vi "VAJ sim.vi"() -> ()   [LabVIEW 2019]
uses:
  <vilib>/Platform/TimedLoop/XDataNode/timing_clust.ctl
  <vilib>/Platform/TimedLoop/XDataNode/nitl_modes.ctl
  <vilib>/Platform/TimedLoop/XDataNode/wakeup.ctl
  <vilib>/platform/TimedLoop/XDataNode/XDataNode.xnode
  <vilib>/Platform/TimedLoop/XDataNode/XDNodeRunTimeDep.lvlib
panel:
  out "Waveform Chart":T1(graph)
  in  "D":dbl
  in  "J":dbl
  in  "A":dbl
  in  "V":dbl
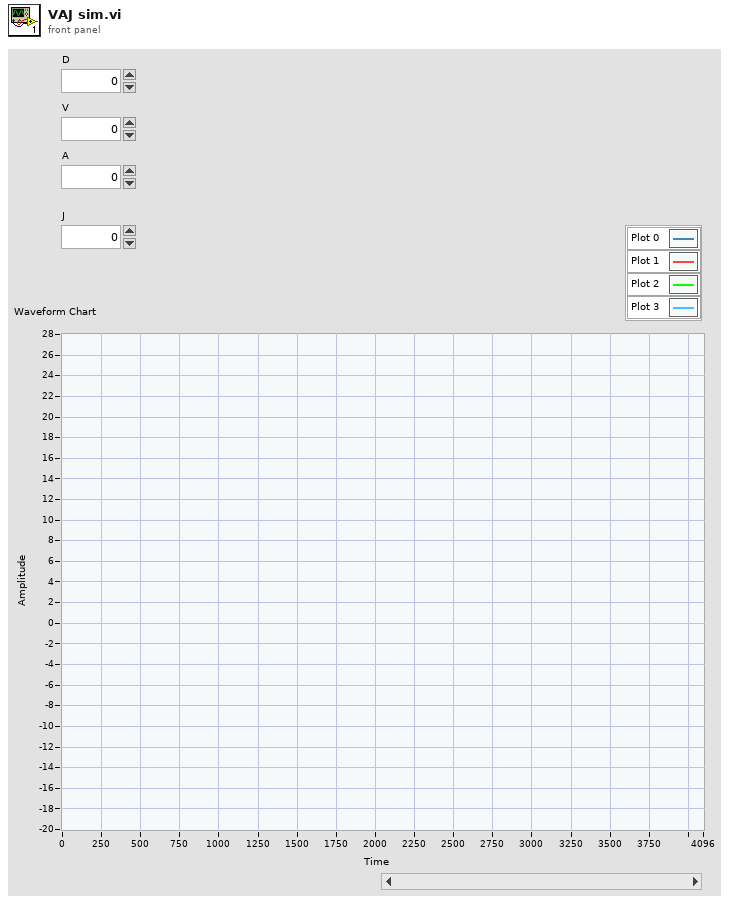
[diagram p1: front panel]
types:
  T1 = cluster{"setpoint":dbl, "integral x(t)":dbl, "integral x(t)":dbl, "integral x(t)":dbl}
  T2 = typedef "XDNodeRunTimeDep.lvlib/timing_clust.ctl" = cluster{"Expected End [f-1]":u64, "Actual End [f-1]":u64, "Finished Late? [f-1]":bool, "Expected End [i-1]":u64, "Actual End [i-1]":u64, "Finished Late? [i-1]":bool, "Expected Start [i]":u64, "Actual Start [i]":u64, "Expected Start [f]":u64, "Actual Start [f]":u64, "Source Name":string, "Structure Name":string, "Period":i64, "Deadline":i64, "Offset":i64, "Start":i64, "Priority":i32, "Timeout":i32, "Mode":T3, "Wakeup Reason":T4, "Error":errorcluster, "Source Type":string, "Secondary Source Type":string, "Global End Time":u64, "Global Start Time":u64, "Frame Duration":u64, "Iteration Duration":u64, "Assigned CPU":i32, "I/O Scan Engine Mode":u32}
  T3 = typedef "XDNodeRunTimeDep.lvlib/nitl_modes.ctl" = enum32{"No Change", "Process missed periods, maintain original phase", "Discard missed periods, maintain original phase", "Process missed periods, ignore original phase", "Discard missed periods, ignore original phase"}
  T4 = typedef "XDNodeRunTimeDep.lvlib/wakeup.ctl" = enum32{"Normal", "Aborted", "Asynchronous wakeup", "Timing source error", "Timed loop error", "Timeout"}
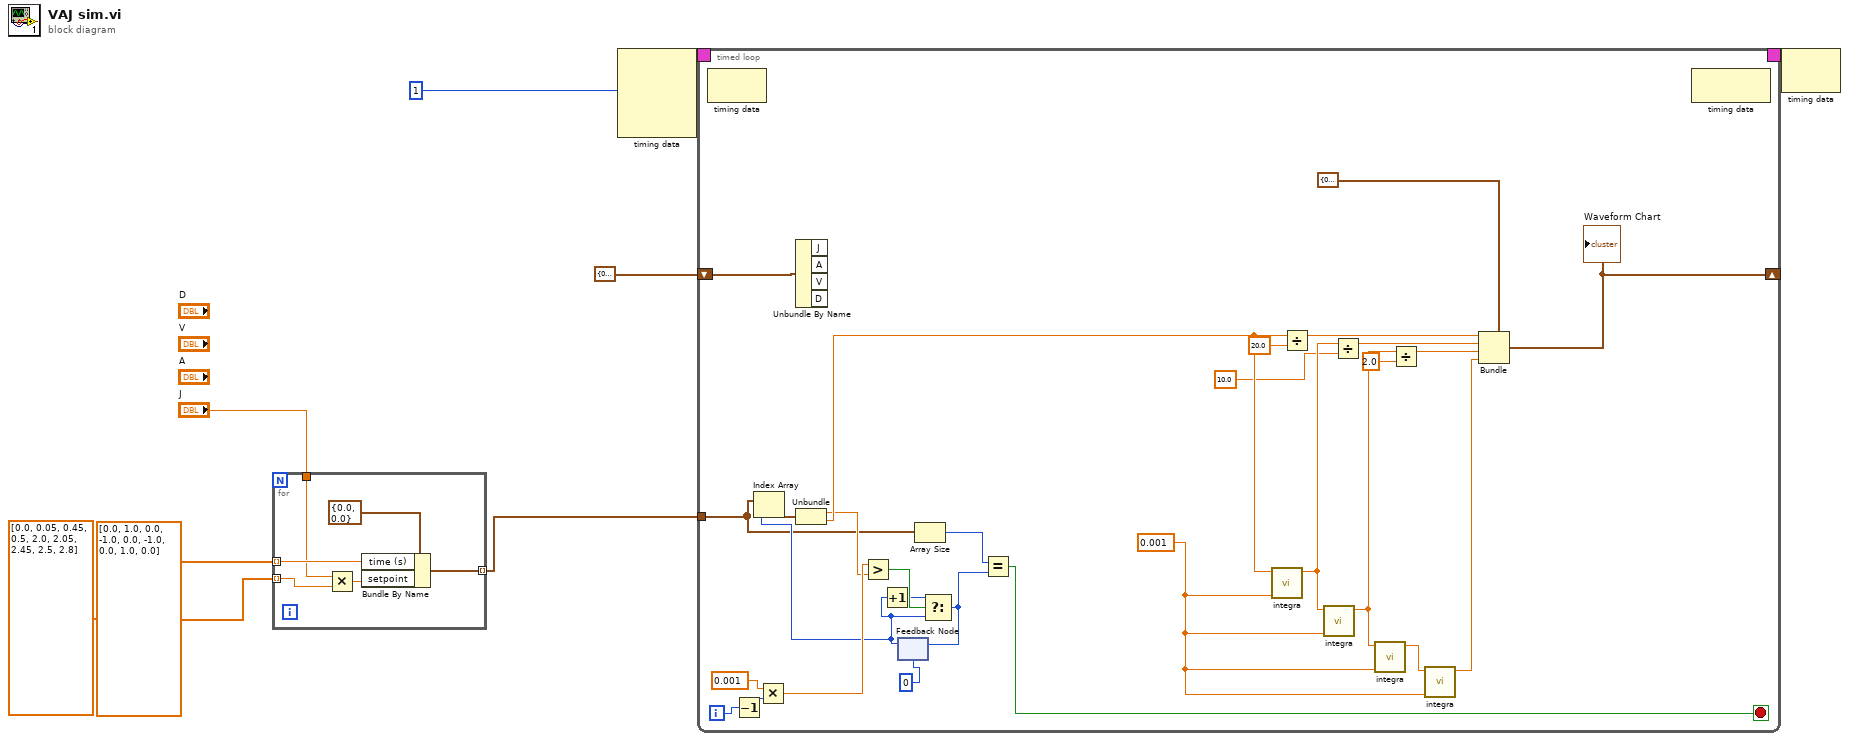
[diagram p0: block diagram]
diagram:
  n1 = for {
    tunnel: dbl[] [0.0, 0.05, 0.45, 0.5, 2.0, 2.05, 2.45, 2.5, 2.8] ("time (s)") -> [w13] mode=indexing
    tunnel: dbl[] [0.0, 1.0, 0.0, -1.0, 0.0, -1.0, 0.0, 1.0, 0.0] ("time (s)") -> [w9] mode=indexing
    tunnel: [w12] -> w3 mode=indexing
    tunnel: "J" -> [w10]
    n2 = Multiply(x=w10, y=w9) -> (x*y=w11:dbl)
    n3 = Bundle By Name(cluster=cluster{"time (s)":dbl, "setpoint":dbl} {"time (s)"=0.0, "setpoint"=0.0}, "time (s)"=w13, "setpoint"=w11) -> (w12:cluster{"time (s)":dbl, "setpoint":dbl})
  }
  n4 = node-c288(i64 1 ("Period")) -> (w8:T2)  [unwired: 3 in]
  n5 = timed-loop {
    timing: w8 -> [_]
    timing-out: [_] -> w7
    tunnel: w3 -> [w29]
    shift-right: [w18] -> _
    shift-left: cluster{"J":dbl, "A":dbl, "V":dbl, "D":dbl} {"J"=0.0, "A"=0.0, "V"=0.0, "D"=0.0} ("cluster") -> [w17]
    i -> [w16]
    stop <- w26 stop-if-true
    w40 = 0.001 ("dt (s)")
    n6 = node-c288() -> ()  [unwired: 1 in, 1 out]
    n7 = Decrement(x=w16) -> (x-1=w15:i32)
    n8 = Multiply(x=0.001, y=w15) -> (x*y=w35:dbl)
    n9 = Unbundle By Name(w17) -> ()  [unwired: 4 out]
    n10 = feedback #1(0) -> (w30:i32)
    n11 = Index Array(array=w29, index=w30) -> (element=w37:cluster{"time (s)":dbl, "setpoint":dbl})
    n12 = Unbundle(w37) -> ("time (s)"=w34:dbl, "setpoint"=w36:dbl)
    n13 = Greater?(x=w35, y=w34) -> (0:w33:bool)
    n14 = Increment(x=w30) -> (x+1=w31:i32)
    n15 = Array Size(array=w29) -> (size(s)=w28:i32)
    n16 = Select(t=w31, s=w33, f=w30) -> (s? t:f=w27:i32)
    n17 = feedback-in #1(w27) -> ()
    n18 = Equal?(x=w28, y=w27) -> (x = y?=w26:bool)
    n19 = call "integra.vi"("period"=w40, "X"=w36) -> ("R"=w43:dbl)  [unwired: 9 in]
    n20 = Divide(x=w36, y=20.0) -> (x/y=w25:dbl)
    n21 = call "integra.vi"("period"=w40, "X"=w43) -> ("R"=w42:dbl)  [unwired: 9 in]
    n22 = Divide(x=w43, y=10.0) -> (x/y=w23:dbl)
    n23 = call "integra.vi"("period"=w40, "X"=w42) -> ("R"=w41:dbl)  [unwired: 9 in]
    n24 = Divide(x=w42, y=2.0) -> (x/y=w21:dbl)
    n25 = call "integra.vi"("period"=w40, "X"=w41) -> ("R"=w39:dbl)  [unwired: 9 in]
    n26 = Bundle(cluster=cluster{"J":dbl, "A":dbl, "V":dbl, "D":dbl} {"J"=0.0, "A"=0.0, "V"=0.0, "D"=0.0}, "J"=w25, "A"=w23, "V"=w21, "D"=w39) -> (w18:cluster{"J":dbl, "A":dbl, "V":dbl, "D":dbl})
    "Waveform Chart" <- w18
    n27 = node-c288() -> ()  [unwired: 1 in, 1 out]
  }
  n28 = node-c288(w7) -> ()  [unwired: 1 out]
